vi "make graph from elements.vi"(10 "toffset":dbl, 11 "elements":T2[](array[typedef])) -> (2 "t offset out":dbl, 3 "graphs":T1)   [LabVIEW 2017]
uses:
  typedefs/reading.ctl
  typedefs/readingType.ctl
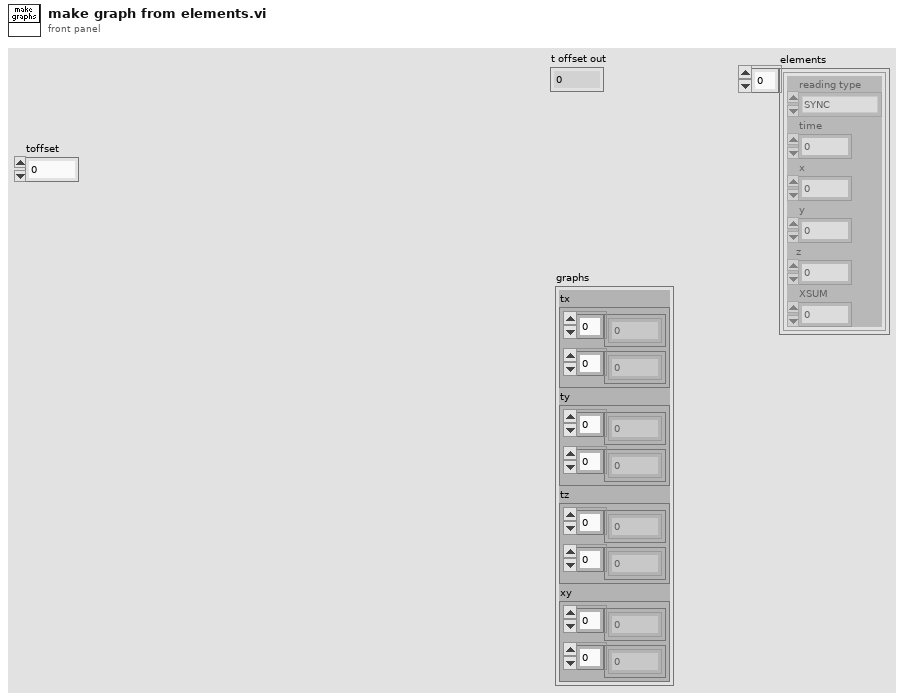
[diagram p1: front panel]
types:
  T1 = cluster{"tx":cluster{dbl[], sgl[]}, "ty":cluster{dbl[], sgl[]}, "tz":cluster{dbl[], sgl[]}, "xy":cluster{sgl[], sgl[]}}
  T2 = typedef "reading.ctl" = cluster{"reading type":T3, "time":fxp<+,48,48>, "x":sgl, "y":sgl, "z":sgl, "XSUM":u8}
  T3 = typedef "readingType.ctl" = enum8{"SYNC", "DETVAL", "COILI", "MAGVEC", "ACCVEC"}
  T4 = cluster{cluster{dbl[], sgl[]}, cluster{dbl[], sgl[]}, cluster{dbl[], sgl[]}, cluster{sgl[], sgl[]}}
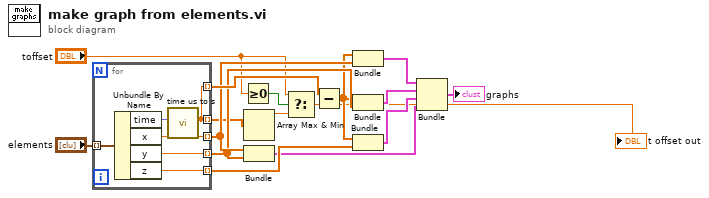
[diagram p0: block diagram]
diagram:
  n1 = for {
    tunnel: "elements" -> [w22] mode=indexing
    tunnel: [w17] -> w15 mode=indexing
    tunnel: [w21] -> w13 mode=indexing
    tunnel: [w20] -> w12 mode=indexing
    tunnel: [w19] -> w14 mode=indexing
    tunnel: [w17] -> w5 mode=indexing
    n2 = Unbundle By Name(w22) -> ("time"=w18:fxp<+,48,48>, "x"=w21:sgl, "y"=w20:sgl, "z"=w19:sgl)
    n3 = call "time us to s.vi"("time (us)"=w18) -> ("time (s)"=w17:dbl)  [unwired: 10 in]
  }
  n4 = Greater Or Equal To 0?(x="toffset") -> (x >= 0?=w4:bool)
  n5 = Array Max & Min(array=w5) -> (max value=w2:dbl)  [unwired: 3 out]
  n6 = Bundle(w13, w12) -> (w8:cluster{sgl[], sgl[]})  [unwired: 1 in]
  n7 = Select(t="toffset", s=w4, f=w2) -> (s? t:f=w1:dbl)
  "t offset out" <- w1
  n8 = Subtract(x=w15, y=w1) -> (x-y=w6:dbl[])
  n9 = Bundle(w6, w13) -> (w11:cluster{dbl[], sgl[]})  [unwired: 1 in]
  n10 = Bundle(w6, w12) -> (w10:cluster{dbl[], sgl[]})  [unwired: 1 in]
  n11 = Bundle(w6, w14) -> (w9:cluster{dbl[], sgl[]})  [unwired: 1 in]
  n12 = Bundle(w11, w10, w9, w8) -> (→"graphs":T4)  [unwired: 1 in]
